vi "DF on PDW.vi"(8 "error in (no error)":errorcluster, 10 "sorted PDWs":T1[](array[typedef]), 11 "device_type in":refnum<class "device_type.lvclass">) -> (0 "error out":errorcluster, 2 "PDWs on channels":cluster{T1[]}[](array[cluster]), 3 "device_type out":refnum<class "device_type.lvclass">)   [LabVIEW 2021, in "device_type.lvclass"]
uses:
  device_type.lvclass
  device_type.lvclass/device_type.ctl
  <vilib>/Analysis/NI_AALBase.lvlib
  <vilib>/Analysis/1siggen.llb/Ramp Pattern by Samples.vi
  pulse_tx_vis/CTL/mode_type.ctl
  pulse_tx_vis/CTL/PDW_lv2.ctl
panel:
  out "time":dbl[](array[numeric])
  out "Ramp Pattern":dbl[](array[numeric])
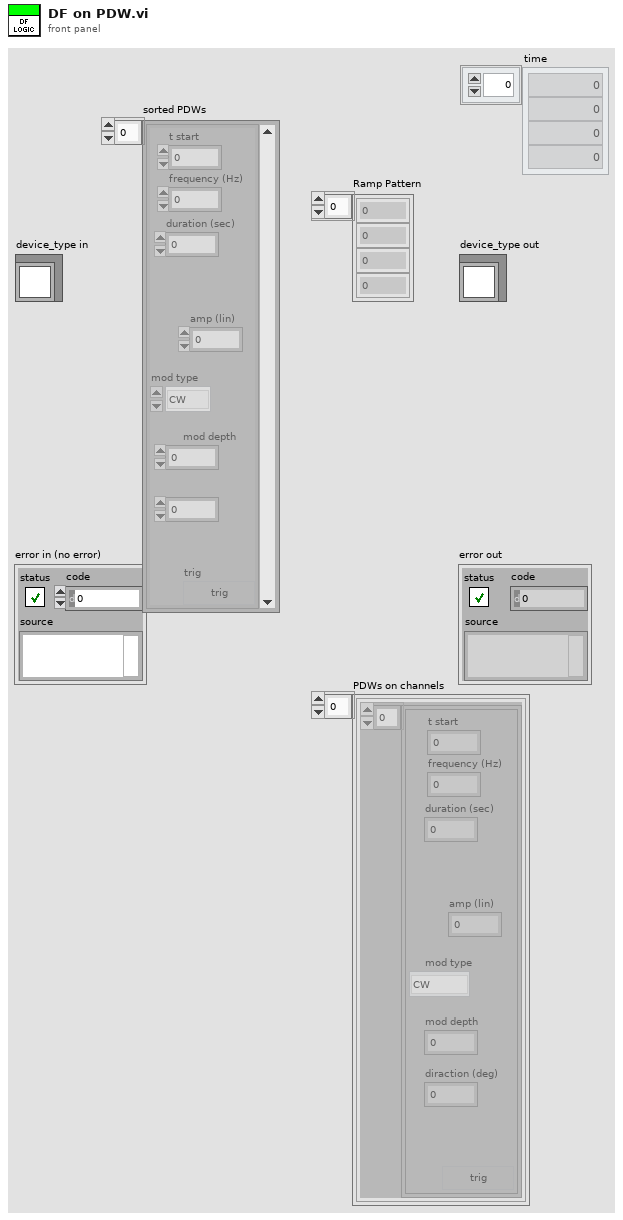
[diagram p1: front panel]
types:
  T1 = typedef "PDW_lv2.ctl" = cluster{"t start":dbl, "frequency (Hz)":dbl, "duration (sec)":dbl, "mod type":T2, "mod depth":dbl, "trig":bool, "amp (lin)":dbl, "diraction (deg)":dbl}
  T2 = typedef "mode_type.ctl" = enum8{"CW", "from memory 1", "NC - cw", "LFM", "BPSK", "QPSK"}
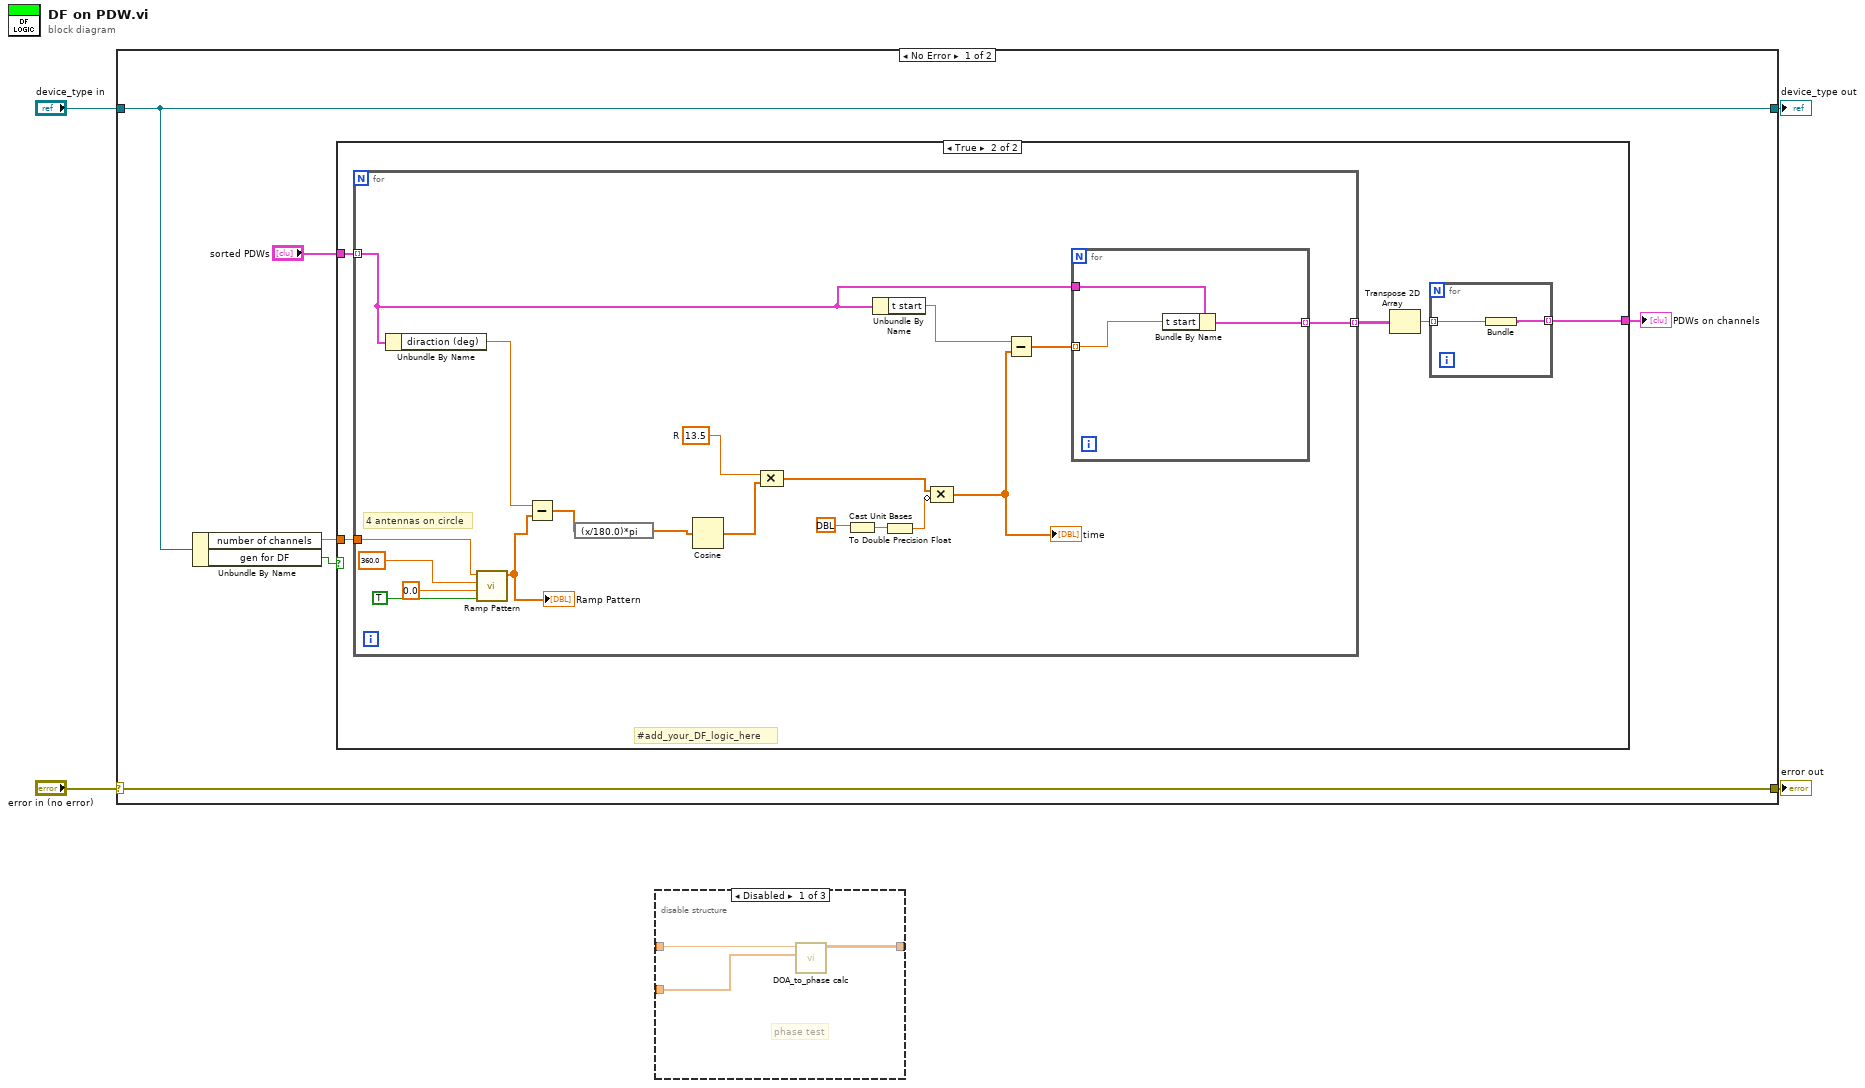
[diagram p0: block diagram]
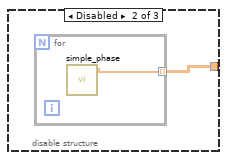
[diagram p2: hidden frame]
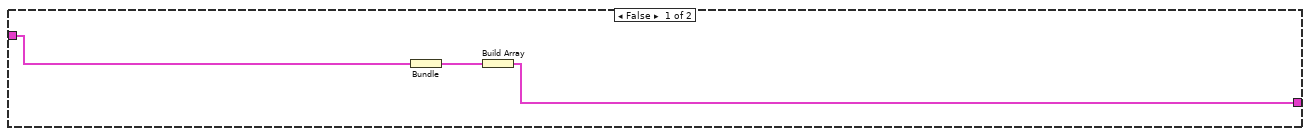
[diagram p4: hidden frame]
diagram:
  n1 = case shown="No Error" "error in (no error)" {
    selector: "error in (no error)" -> [w10 w44]
    tunnel: [w10 w44] -> w3
    tunnel: [w9 w43] -> w1
    tunnel: "device_type in" -> [w9 w43]
    frame No Error {
      n2 = Unbundle By Name(w9) -> ("number of channels"=w7:dbl, "gen for DF"=w6:bool)
      n3 = case shown="True" w6 {
        tunnel: "sorted PDWs" -> [w13 w18]
        tunnel: w7 -> [_ w15]
        tunnel: [w11 w14] -> w5
        frame False {
          n4 = Bundle("sorted PDWs"=w13) -> (w12:cluster{"sorted PDWs ":T1[]})  [unwired: 1 in]
          n5 = Build Array(w12) -> (w11:cluster{"sorted PDWs ":T1[]}[])
        }
        frame True {
          # "#add_your_DF_logic_here"
          n6 = for {
            tunnel: w18 -> [w22] mode=indexing
            tunnel: [w24] -> w17 mode=indexing
            tunnel: w15 -> [w23]
            w37 = 13.5  # R
            # "4 antennas on circle"
            n7 = Unbundle By Name(w22) -> ("diraction (deg)"=w21:dbl)
            n8 = call-poly <vilib>:"Ramp Pattern.vi"("exclude end?"=TRUE, "start"=0.0, "end"=360.0, "samples"=w23) -> ("Ramp Pattern"=w35:dbl[])  [unwired: 6 in, 1 out]
            "Ramp Pattern" <- w35
            n9 = Subtract(x=w21, y=w35) -> (x-y=w33:dbl[])
            n10 = expression code="(x/180.0)*pi" ("degrees to radians")(w33) -> (w32:dbl[])
            n11 = Cosine(x=w32) -> (cos(x)=w36:dbl[])
            n12 = Compound Arithmetic op=MULTIPLY(w37, w36) -> (w29:dbl[])
            n13 = Cast Unit Bases(0:ext[unit] 299792458.0) -> (2:w30:ext)  [unwired: 1 in]
            n14 = Unbundle By Name(w22) -> ("t start"=w27:dbl)
            n15 = To Double Precision Float(number=w30) -> (double precision float=w28:dbl)
            n16 = Compound Arithmetic op=MULTIPLY(w29, invert w28) -> (w26:dbl[])
            "time" <- w26
            n17 = Subtract(x=w27, y=w26) -> (x-y=w25:dbl[])
            n18 = for {
              tunnel: w25 -> [w41] mode=indexing
              tunnel: w22 -> [w42]
              tunnel: [w40] -> w24 mode=indexing
              n19 = Bundle By Name(cluster=w42, "t start"=w41) -> (w40:T1)
            }
          }
          n20 = Transpose 2D Array(2D array=w17) -> (transposed array=w16:T1[][])
          n21 = for {
            tunnel: w16 -> [w20] mode=indexing
            tunnel: [w19] -> w14 mode=indexing
            n22 = Bundle(w20) -> (w19:cluster{T1[]})  [unwired: 1 in]
          }
        }
      }
      "PDWs on channels" <- w5
    }
    frame Error {
    }
  }
  "error out" <- w3
  "device_type out" <- w1
  n23 = disable-structure shown="Disabled" {
    disable-tunnel: _ -> [w47 _ _]
    disable-tunnel: _ -> [w46 _ _]
    disable-tunnel: [w45 w48 _] -> _
    frame Disabled {
      # "phase test"
      n24 = call "DOA_to_phase calc.vi"("f set (Hz)"=w46, "DOA (deg)"=w47) -> ("phase (rad)"=w45:dbl[][])  [unwired: 9 in]
    }
    frame Disabled {
      n25 = for {
        tunnel: [w49] -> w48 mode=indexing
        n26 = call "simple_phase.vi"() -> ("simple phase"=w49:dbl[])  [unwired: 11 in]
      }
    }
    frame Enabled {
    }
  }
